vi "W9EO82,FBO8PP_4 (2).vi"() -> ()   [LabVIEW 2021]
uses:
  <vilib>/Analysis/NI_AALPro.lvlib
panel:
  out "number":i64
  out "Array 2":i64[](array[numeric])
  out "Histogram":i32[](array[numeric])
  out "Histogram Graph":T1(graph)
  in  "Gomb":bool
  out "Boolean":bool
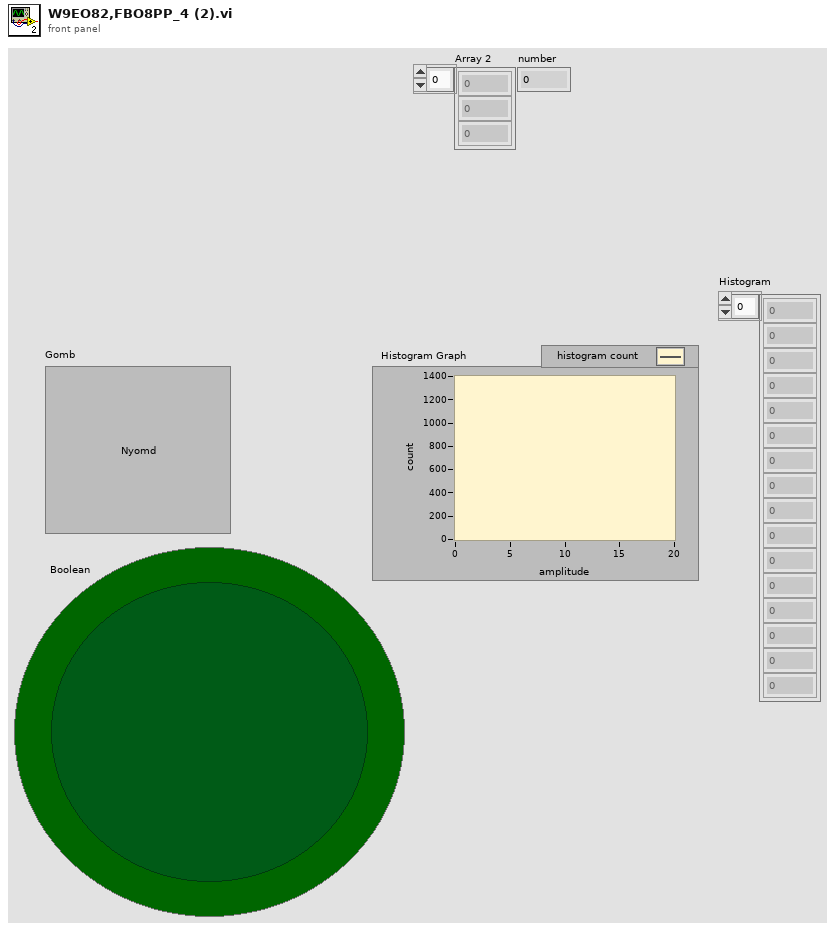
[diagram p1: front panel]
types:
  T1 = cluster{"X Values":dbl[], "Histogram: h(x)":i32[]}
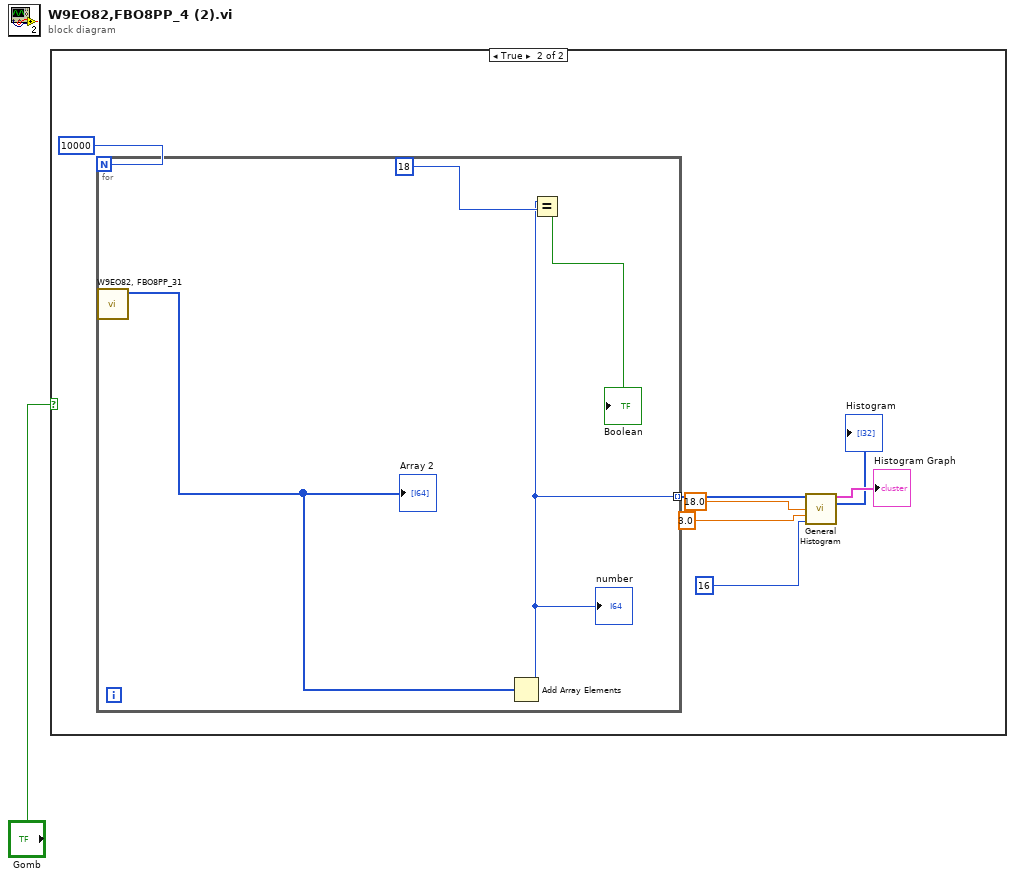
[diagram p0: block diagram]
diagram:
  n1 = case shown="True" "Gomb" {
    frame False {
    }
    frame True {
      n2 = for {
        N: 10000 -> [_]
        tunnel: [w9] -> w3 mode=indexing
        n3 = call "W9EO82, FBO8PP_31.vi"() -> ("Array"=w11:i64[])  [unwired: 11 in]
        "Array 2" <- w11
        n4 = Add Array Elements(numeric array=w11) -> (sum=w9:i64)
        "number" <- w9
        n5 = Equal?(x=w9, y=18) -> (x = y?=→"Boolean":bool)
      }
      n6 = call <vilib>:"General Histogram.vi"("X"=w3, "max"=18.0, "min"=3.0, "# bins"=16) -> ("Histogram Graph"=→"Histogram Graph":T1, "Histogram"=→"Histogram":i32[])  [unwired: 7 in, 3 out]
    }
  }
